vi "GetDiagramUIDs.vi"(6 "error in":errorcluster, 9 "Structure in":refnum<class "Structure.lvclass">) -> (0 "error out":errorcluster, 3 "Structure out":refnum<class "Structure.lvclass">, 4 "diagrams":i32[](array[numeric]))   [LabVIEW 2014, in "Raspberry Pi Compatible Compiler for LabVIEW.lvlib" / "Structure.lvclass"]
uses:
  Structure.lvclass
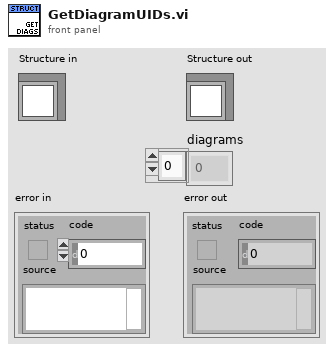
[diagram p1: front panel]
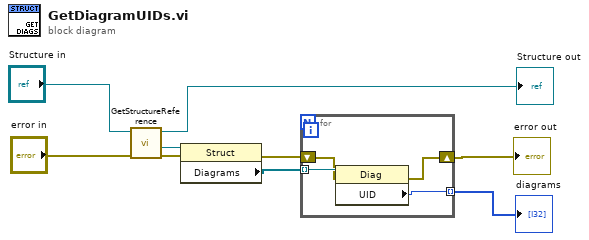
[diagram p0: block diagram]
diagram:
  n1 = call "GetStructureReference.vi"("error in"="error in", "Structure in"="Structure in") -> ("error out"=w6:errorcluster, "reference out"=w7:refnum<vi>, "Structure out"=→"Structure out":refnum<class "Structure.lvclass">)  [unwired: 7 in]
  n2 = property class="Struct"(reference=w7, error in=w6) -> (error out=w5:errorcluster, "Diagrams"=w4:refnum<vi>[])  [unwired: 1 out]
  n3 = for {
    shift-right: [w11] -> w2
    shift-left: w5 -> [w12]
    tunnel: w4 -> [w13] mode=indexing
    tunnel: [w10] -> w1 mode=indexing
    n4 = property class="Diag"(reference=w13, error in=w12) -> (error out=w11:errorcluster, "UID"=w10:i32)  [unwired: 1 out]
  }
  "error out" <- w2
  "diagrams" <- w1
